vi "myRIO_BRig_Host_TCP_parseCmd_analogInput.vi"(10 "input_countCmd":i32, 11 "input_strCmd":string) -> (0 "output_ai1":i32, 1 "output_ai0":i32, 3 "output_haveAnalogInput":bool)   [LabVIEW 2014]
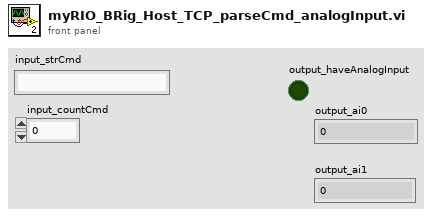
[diagram p1: front panel]
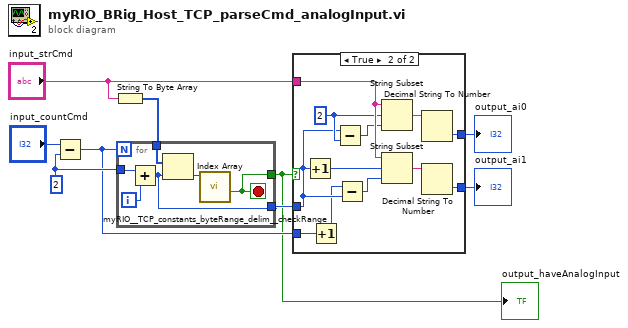
[diagram p0: block diagram]
diagram:
  w8 = 2 ("y")
  n1 = Subtract(x="input_countCmd", y=w8) -> (x-y=w4:i32)
  n2 = String To Byte Array(string="input_strCmd") -> (unsigned byte array=w7:u8[])
  n3 = for {
    N: w4 -> [_]
    tunnel: w8 -> [w14]
    tunnel: w7 -> [w12]
    tunnel: [w11] -> w6
    tunnel: [w10] -> w3
    i -> [w13]
    stop <- w10 stop-if-true
    n4 = Add(x=w14, y=w13) -> (x+y=w11:i32)
    n5 = Index Array(array=w12, index=w11) -> (element=w15:u8)
    n6 = call "myRIO__TCP_constants_byteRange_delim__checkRange.vi"("input_byte"=w15) -> ("output_delim_1"=w10:bool)  [unwired: 9 in, 1 out]
  }
  "output_haveAnalogInput" <- w3
  n7 = case shown="True" w3 {
    tunnel: w6 -> [_ w18]
    tunnel: "input_strCmd" -> [_ w27]
    tunnel: w4 -> [_ w17]
    tunnel: [_ w20] -> w2
    tunnel: [_ w19] -> w1
    frame False {
    }
    frame True {
      w26 = 2 ("offset (0)")
      n8 = Increment(x=w18) -> (x+1=w24:i32)
      n9 = Increment(x=w17) -> (x+1=w16:i32)
      n10 = Subtract(x=w18, y=w26) -> (x-y=w25:i32)
      n11 = Subtract(x=w16, y=w18) -> (x-y=w23:i32)
      n12 = String Subset(string=w27, offset (0)=w26, length (rest)=w25) -> (substring=w22:string)
      n13 = String Subset(string=w27, offset (0)=w24, length (rest)=w23) -> (substring=w21:string)
      n14 = Decimal String To Number(string=w22) -> (number=w20:i32)  [unwired: 2 in, 1 out]
      n15 = Decimal String To Number(string=w21) -> (number=w19:i32)  [unwired: 2 in, 1 out]
    }
  }
  "output_ai0" <- w2
  "output_ai1" <- w1
